vi "Example Threshold - WeightReached Callback.vi"(4 "WeightReached":refnum<user-event>, 5 "Event Data":cluster{"sender":refnum<k24>, "weight":i32}, 6 "Control Ref":refnum<k24>, 7 "Event Common Data":T1) -> ()   [LabVIEW 2013]
uses:
  C:/tf/play/labview/Tinkerforge.dll
  Tinkerforge.dll
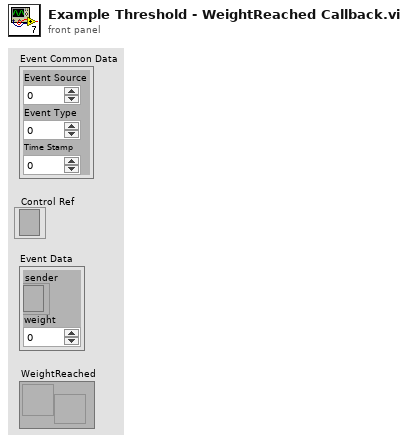
[diagram p1: front panel]
types:
  T1 = cluster{"Event Source":i32, "Event Type":u32, "Time Stamp":u32}
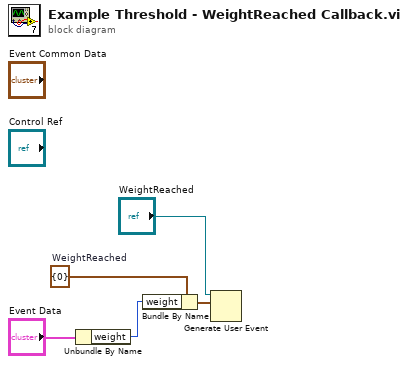
[diagram p0: block diagram]
diagram:
  w4 = cluster{"weight":i32} {"weight"=0}  # WeightReached
  n1 = Unbundle By Name("Event Data") -> ("weight"=w3:i32)
  n2 = Bundle By Name(cluster=w4, "weight"=w3) -> (w2:cluster{"weight":i32})
  n3 = Generate User Event(user event="WeightReached", event data cluster=w2) -> ()  [unwired: 2 in, 2 out]
